vi "zad1.vi"() -> ()   [LabVIEW 2017]
panel:
  in  "stop":bool
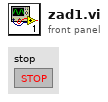
[diagram p1: front panel]
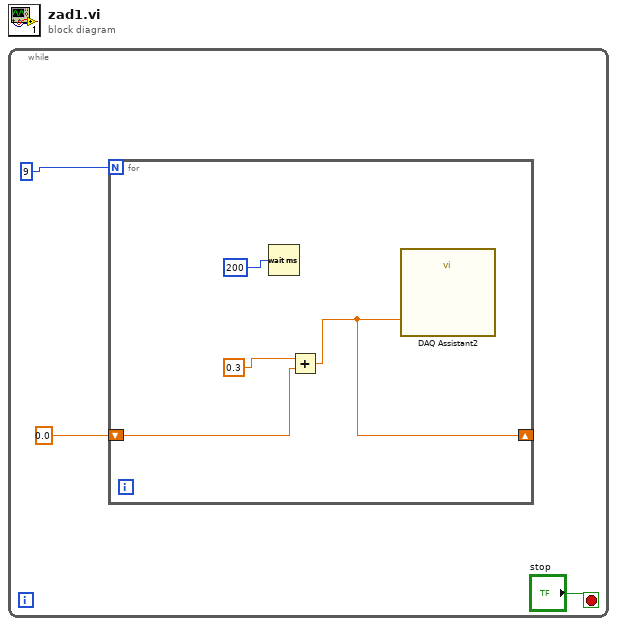
[diagram p0: block diagram]
diagram:
  n1 = while {
    stop <- "stop" stop-if-true
    n2 = for {
      N: 9 -> [_]
      shift-right: [w5] -> _
      shift-left: 0.0 -> [w7]
      n3 = Wait (ms)(milliseconds to wait=200) -> ()  [unwired: 1 out]
      n4 = Add(x=0.3, y=w7) -> (x+y=w5:dbl)
      n5 = call "DAQ Assistant2"("data"=w5) -> ()  [unwired: 17 in, 2 out]
    }
  }
